vi "2_3.vi"() -> ()   [LabVIEW 2010]
uses:
  конт.ctl
panel:
  out "Відсортована таблиця у порядку спадання":string[][](table)
  in  "stop":bool
  in  "Рік":bool
  in  "По батькові":bool
  in  "Ім'я":bool
  in  "Фамілія":bool
  in  "Відсортована таблиця у порядку спадання":string[][](table)
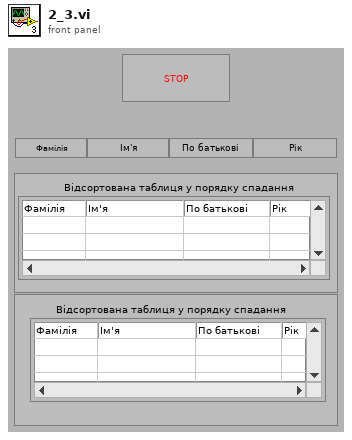
[diagram p1: front panel]
types:
  T1 = typedef "конт.ctl" = enum16{"сортування", "стоп"}
  T2 = cluster{"[0]":string, "[1]":string, "[2]":string, "[3]":string, "[4]":string, "[5]":string, "[6]":string, "[7]":string, "[8]":string}
  T3 = cluster{"[0]":string, "[1]":string, "[2]":string, "[3]":string, "[4]":string, "[5]":string, "[6]":string, "[7]":string, "[8]":string}[]
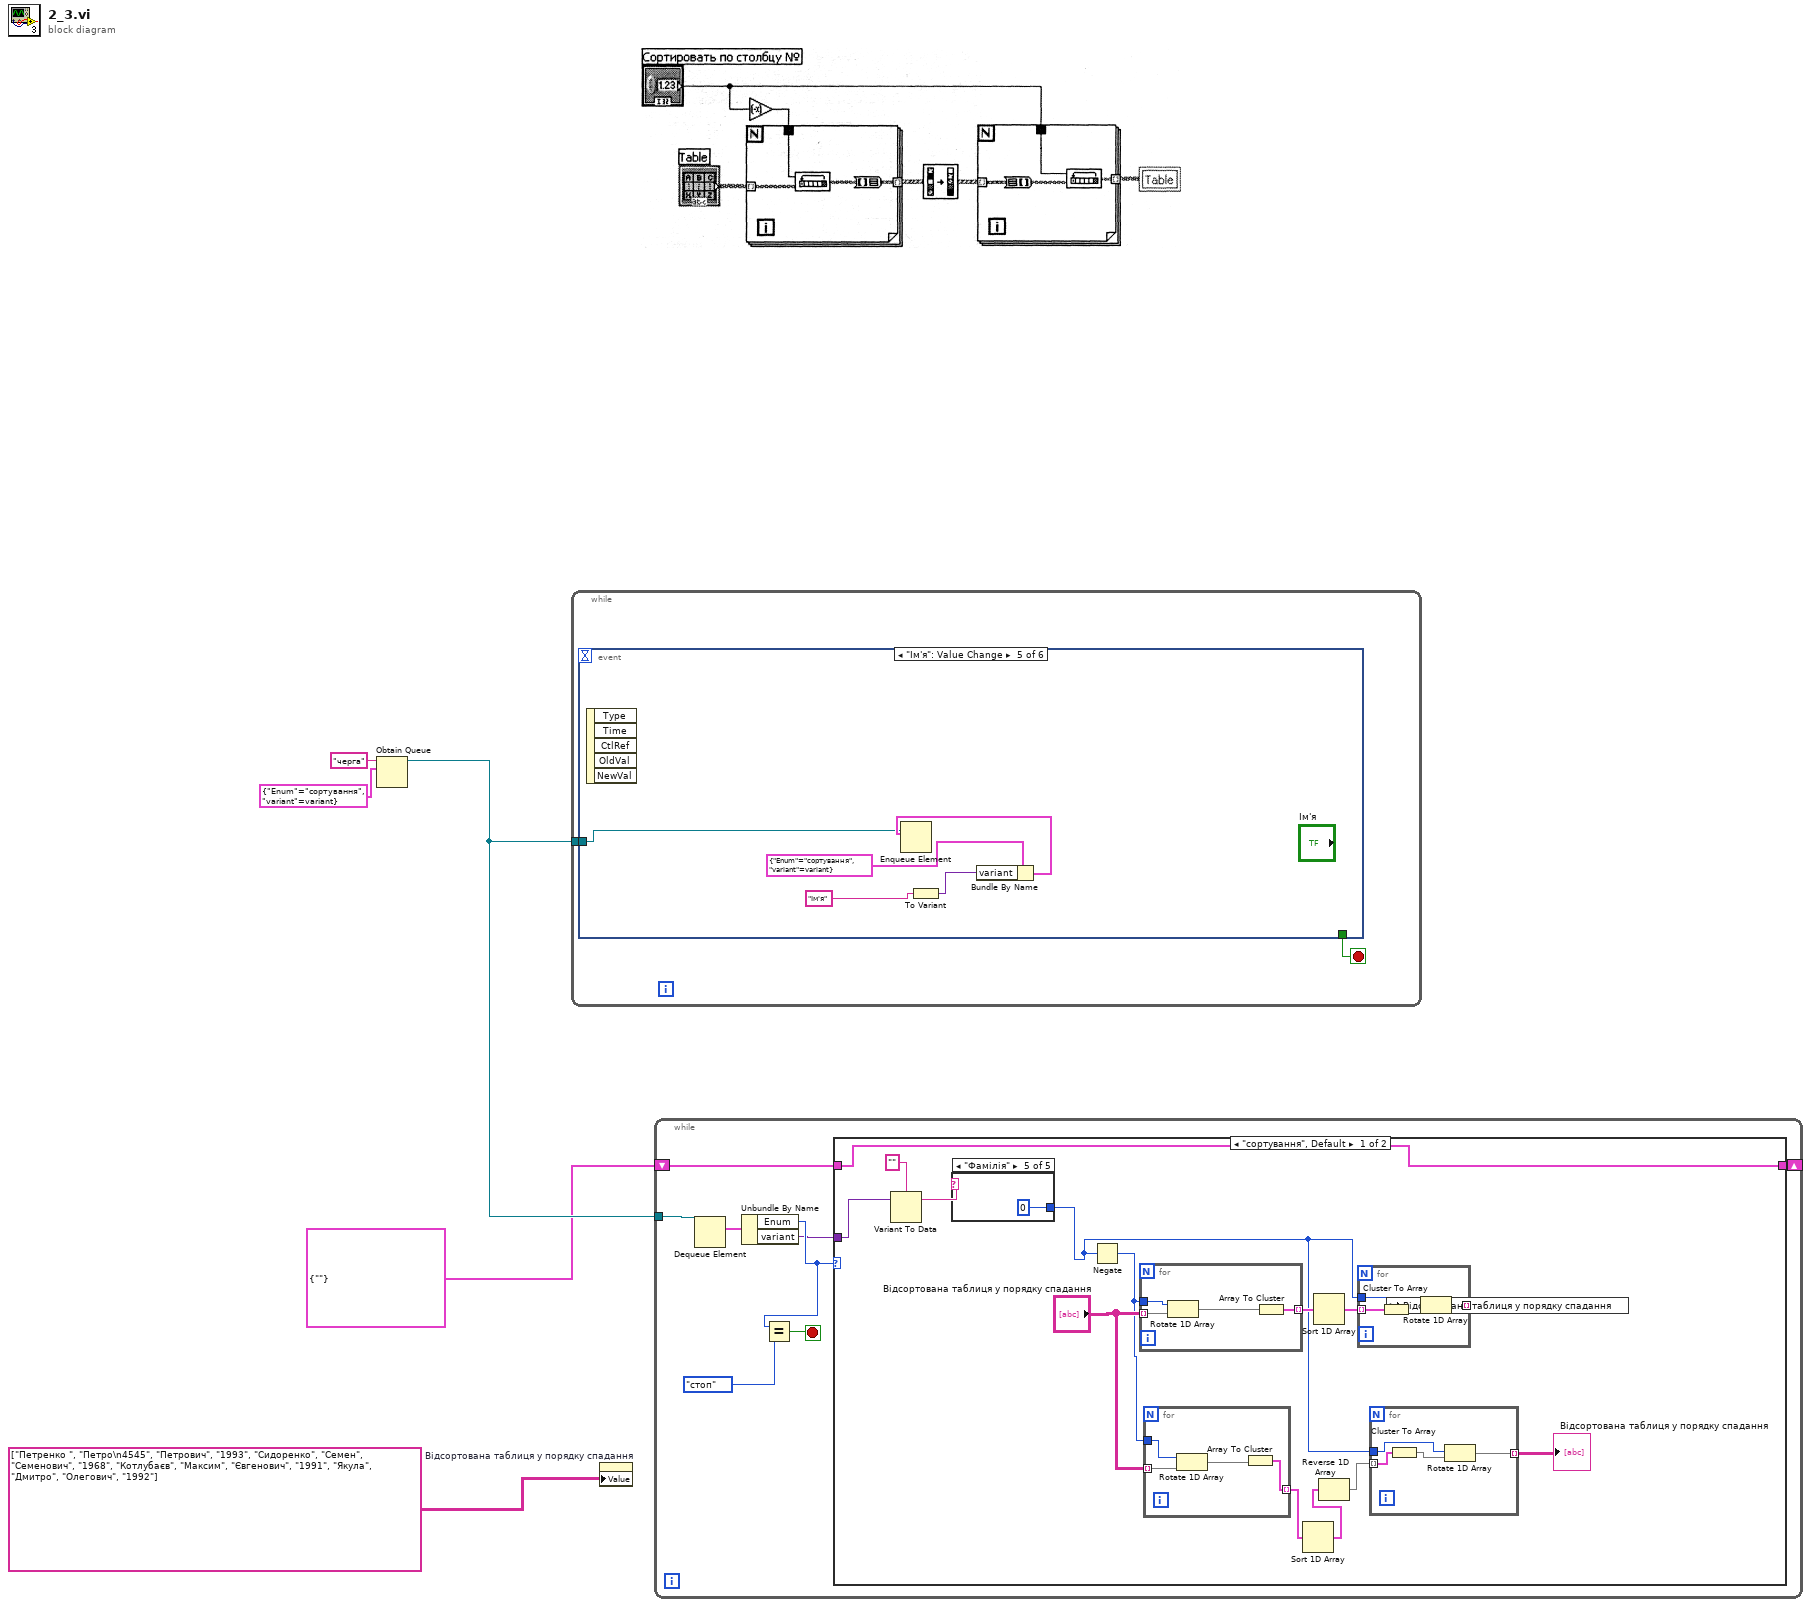
[diagram p0: block diagram]
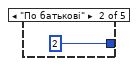
[diagram p3: hidden frame]
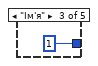
[diagram p4: hidden frame]
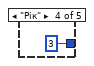
[diagram p5: hidden frame]
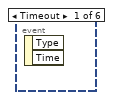
[diagram p7: hidden frame]
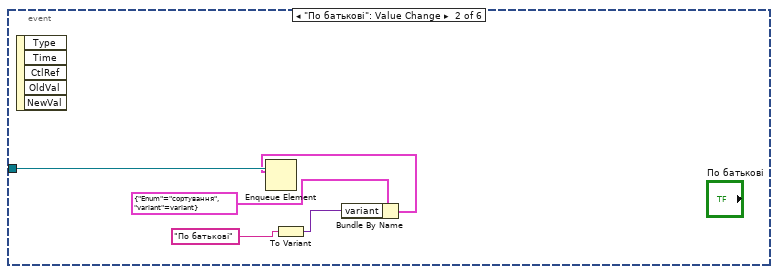
[diagram p8: hidden frame]
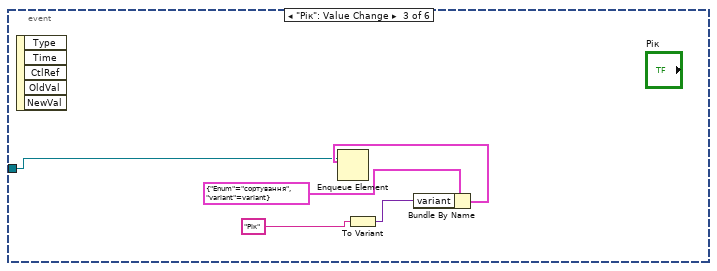
[diagram p9: hidden frame]
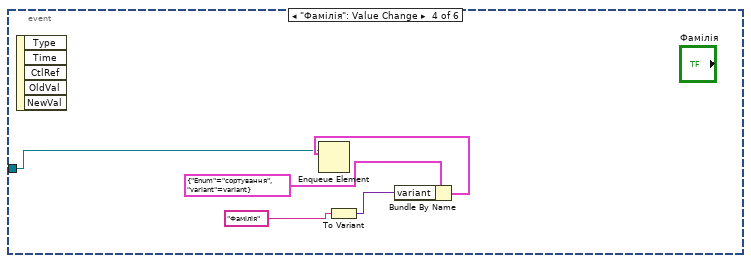
[diagram p10: hidden frame]
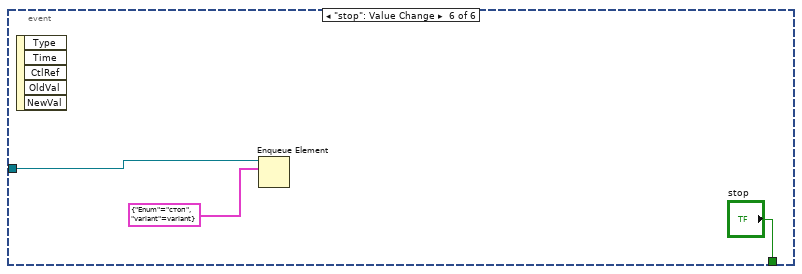
[diagram p11: hidden frame]
diagram:
  n1 = Obtain Queue(name (unnamed)="черга", element data type=cluster{"Enum":T1, "variant":variant} {"Enum"=enum."сортування", "variant"=variant}) -> (queue out=w3:refnum<queue>)  [unwired: 3 in, 2 out]
  n2 = while {
    tunnel: w3 -> [w6]
    stop <- w7 stop-if-true
    n3 = event shown="[4] \"Ім'я\": Value Change" {
      selector: _ -> [_ _ _ _ _ _]
      dyn-events: _ -> [_ _ _ _ _ _]
      timeout: _ -> [_ _ _ _ _ _]
      tunnel: [_ _ _ _ _ "stop"] -> w7
      tunnel: w6 -> [_ w12 w13 w18 w23 w28]
      event Timeout {
        n4 = event-data() -> ()  [unwired: 1 in, 2 out]
      }
      event "По батькові": Value Change {
        n5 = event-data() -> ()  [unwired: 1 in, 5 out]
        n6 = To Variant(anything="По батькові") -> (Variant=w8:variant)
        n7 = Bundle By Name(cluster=cluster{"Enum":T1, "variant":variant} {"Enum"=enum."сортування", "variant"=variant}, "variant"=w8) -> (w10:cluster{"Enum":T1, "variant":variant})
        n8 = Enqueue Element(queue=w12, element=w10) -> ()  [unwired: 2 in, 3 out]
      }
      event "Рік": Value Change {
        n9 = event-data() -> ()  [unwired: 1 in, 5 out]
        n10 = To Variant(anything="Рік") -> (Variant=w14:variant)
        n11 = Bundle By Name(cluster=cluster{"Enum":T1, "variant":variant} {"Enum"=enum."сортування", "variant"=variant}, "variant"=w14) -> (w16:cluster{"Enum":T1, "variant":variant})
        n12 = Enqueue Element(queue=w13, element=w16) -> ()  [unwired: 2 in, 3 out]
      }
      event "Фамілія": Value Change {
        n13 = event-data() -> ()  [unwired: 1 in, 5 out]
        n14 = To Variant(anything="Фамілія") -> (Variant=w19:variant)
        n15 = Bundle By Name(cluster=cluster{"Enum":T1, "variant":variant} {"Enum"=enum."сортування", "variant"=variant}, "variant"=w19) -> (w21:cluster{"Enum":T1, "variant":variant})
        n16 = Enqueue Element(queue=w18, element=w21) -> ()  [unwired: 2 in, 3 out]
      }
      event "Ім'я": Value Change {
        n17 = event-data() -> ()  [unwired: 1 in, 5 out]
        n18 = To Variant(anything="Ім'я") -> (Variant=w24:variant)
        n19 = Bundle By Name(cluster=cluster{"Enum":T1, "variant":variant} {"Enum"=enum."сортування", "variant"=variant}, "variant"=w24) -> (w26:cluster{"Enum":T1, "variant":variant})
        n20 = Enqueue Element(queue=w23, element=w26) -> ()  [unwired: 2 in, 3 out]
      }
      event "stop": Value Change {
        n21 = event-data() -> ()  [unwired: 1 in, 5 out]
        n22 = Enqueue Element(queue=w28, element=cluster{"Enum":T1, "variant":variant} {"Enum"=enum."стоп", "variant"=variant}) -> ()  [unwired: 2 in, 3 out]
      }
    }
  }
  n23 = property on="Відсортована таблиця у порядку спадання" class="Tbl (strict)"("Value"=string[][] [["Петренко ", "Петро\n4545", "Петрович", "1993"], ["Сидоренко", "Семен", "Семенович", "1968"], ["Котлубаєв", "Максим", "Євгенович", "1991"], ["Якула", "Дмитро", "Олегович", "1992"]] ("Table")) -> ()  [unwired: 2 in, 2 out]
  n24 = while {
    tunnel: w3 -> [w38]
    shift-right: [w32] -> _
    shift-left: cluster{string} {""} -> [w33]
    stop <- w35 stop-if-true
    n25 = Dequeue Element(queue=w38) -> (element=w37:cluster{"Enum":T1, "variant":variant})  [unwired: 2 in, 3 out]
    n26 = Unbundle By Name(w37) -> ("Enum"=w36:T1, "variant"=w34:variant)
    n27 = Equal?(x=w36, y=конт."стоп" ("Enum")) -> (x = y?=w35:bool)
    n28 = case shown="\"сортування\", Default" w36 {
      tunnel: w34 -> [w52 _]
      tunnel: w33 -> [w50 w73]
      tunnel: [w50 w73] -> w32
      frame "сортування", Default {
        n29 = Variant To Data(Variant=w52, type="") -> (data=w49:string)  [unwired: 1 in, 1 out]
        n30 = case shown="\"Фамілія\"" w49 {
          tunnel: [_ 2 1 3 0] -> w43
          frame "False", Default {
          }
          frame "По батькові" {
          }
          frame "Ім'я" {
          }
          frame "Рік" {
          }
          frame "Фамілія" {
          }
        }
        n31 = Negate(x=w43) -> (-x=w44:i32)
        n32 = for {
          tunnel: w44 -> [w68]
          tunnel: "Відсортована таблиця у порядку спадання" -> [w65] mode=indexing
          tunnel: [w66] -> w48 mode=indexing
          n33 = Rotate 1D Array(1:w65, 2:w68) -> (0:w67:string[])
          n34 = Array To Cluster(array=w67) -> (cluster=w66:T2)
        }
        n35 = for {
          tunnel: "Відсортована таблиця у порядку спадання" -> [w60] mode=indexing
          tunnel: w44 -> [w57]
          tunnel: [w58] -> w41 mode=indexing
          n36 = Rotate 1D Array(1:w60, 2:w57) -> (0:w59:string[])
          n37 = Array To Cluster(array=w59) -> (cluster=w58:T2)
        }
        n38 = Sort 1D Array(array=w41) -> (sorted array=w40:T3)
        n39 = Sort 1D Array(array=w48) -> (sorted array=w47:T3)
        n40 = Reverse 1D Array(array=w40) -> (reversed array=w42:T3)
        n41 = for {
          tunnel: w43 -> [w62]
          tunnel: w47 -> [w64] mode=indexing
          tunnel: [w61] -> w46 mode=indexing
          n42 = Cluster To Array(cluster=w64) -> (array=w63:string[])
          n43 = Rotate 1D Array(1:w63, 2:w62) -> (0:w61:string[])
        }
        n44 = for {
          tunnel: w43 -> [w53]
          tunnel: w42 -> [w56] mode=indexing
          tunnel: [w54] -> w39 mode=indexing
          n45 = Cluster To Array(cluster=w56) -> (array=w55:string[])
          n46 = Rotate 1D Array(1:w55, 2:w53) -> (0:w54:string[])
        }
        "Відсортована таблиця у порядку спадання" <- w39
        n47 = local write "Відсортована таблиця у порядку спадання"(w46) -> ()
      }
      frame "стоп" {
      }
    }
  }
